vi "Week 3 Practical - CPitcel.vi"() -> ()   [LabVIEW 2018]
panel:
  out "Prime Result":string
  in  "Stop Operation":bool
  in  "Operation":string(combo)="Select Op"
  in  "Operand X":dbl
  in  "Operand Y":dbl
  out "Result":dbl
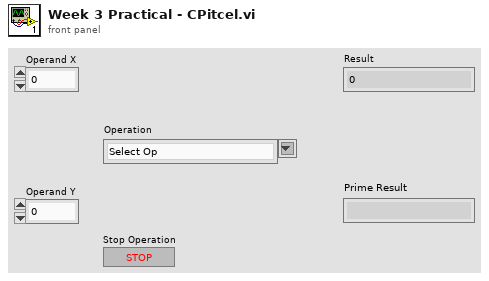
[diagram p1: front panel]
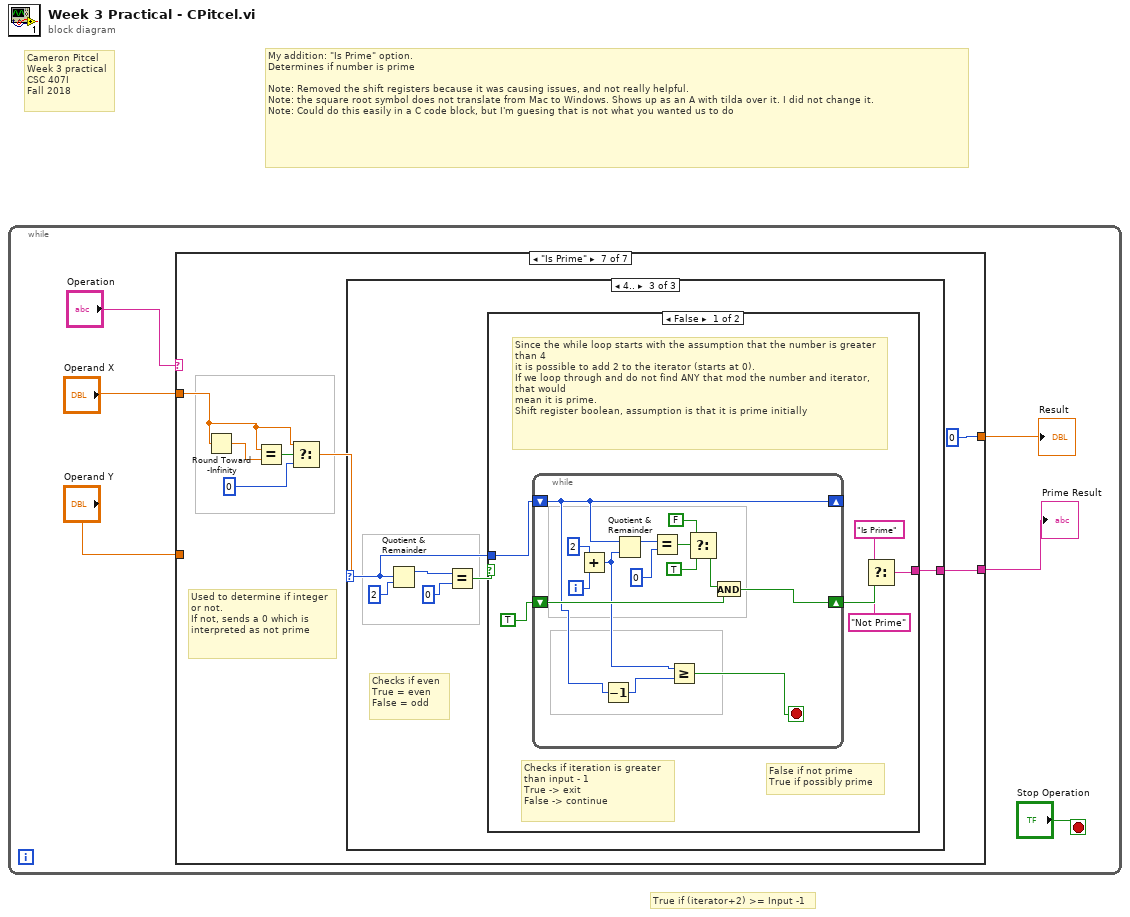
[diagram p0: block diagram]
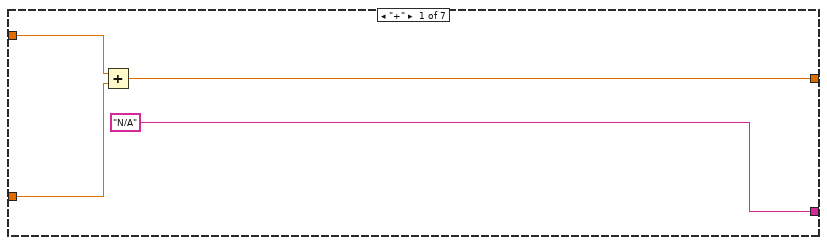
[diagram p2: hidden frame]
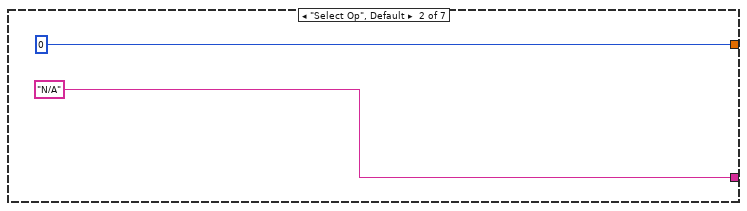
[diagram p3: hidden frame]
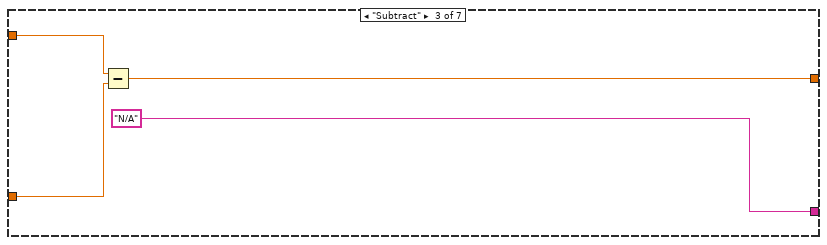
[diagram p4: hidden frame]
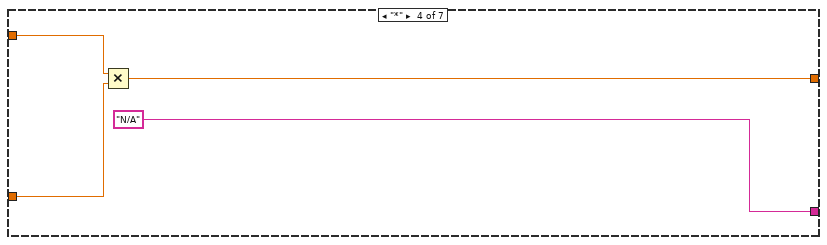
[diagram p5: hidden frame]
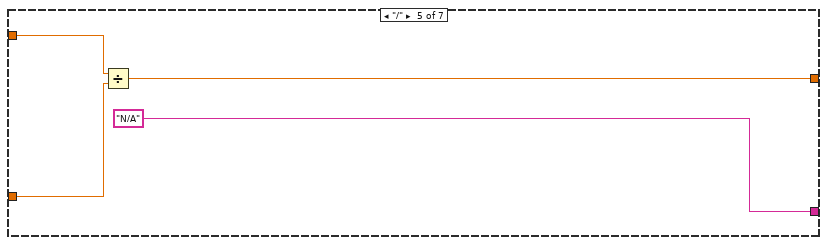
[diagram p6: hidden frame]
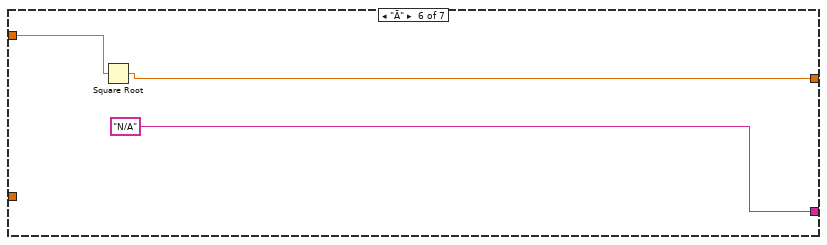
[diagram p7: hidden frame]
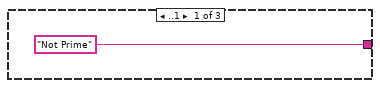
[diagram p8: hidden frame]
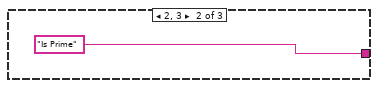
[diagram p9: hidden frame]
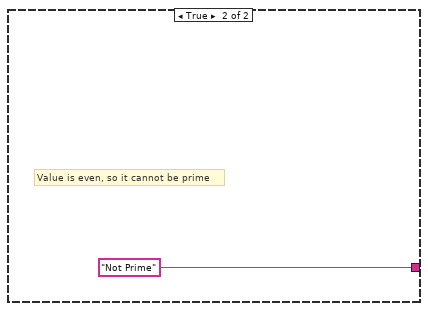
[diagram p10: hidden frame]
diagram:
  # "Cameron Pitcel\nWeek 3 practical\nCSC 407I\nFall 2018"
  # "True if (iterator+2) >= Input -1"
  # "My addition: \"Is Prime\" option.\nDetermines if number is prime\n\nNote: Removed the shift registers because it was causing issues, and not really helpful.\nNote: the square root symbol does not translate from Mac to Windows. Shows up as an A with tilda over it. I did not change it.\nNote: Could do this easily in a C code block, but I'm guesing that is not what you wanted us to do"
  n1 = while {
    stop <- "Stop Operation" stop-if-true
    n2 = case shown="\"Is Prime\"" "Operation" {
      tunnel: "Operand Y" -> [w9 _ w15 w19 w23 _ _]
      tunnel: "Operand X" -> [w10 _ w16 w20 w24 w27 w30]
      tunnel: [w8 0 w14 w18 w22 w26 0] -> w2
      tunnel: ["N/A" "N/A" "N/A" "N/A" "N/A" "N/A" w28] -> w1
      frame "+" {
        n3 = Add(x=w10, y=w9) -> (x+y=w8:dbl)
      }
      frame "Select Op", Default {
      }
      frame "Subtract" {
        n4 = Subtract(x=w16, y=w15) -> (x-y=w14:dbl)
      }
      frame "*" {
        n5 = Multiply(x=w20, y=w19) -> (x*y=w18:dbl)
      }
      frame "/" {
        n6 = Divide(x=w24, y=w23) -> (x/y=w22:dbl)
      }
      frame "Ã" {
        n7 = Square Root(x=w27) -> (sqrt(x)=w26:dbl)
      }
      frame "Is Prime" {
        # "Used to determine if integer or not.\nIf not, sends a 0 which is interpreted as not prime"
        n8 = Round Toward -Infinity(1:w30) -> (0:w33:dbl)
        n9 = Equal?(x=w30, y=w33) -> (x = y?=w31:bool)
        n10 = Select(t=w30, s=w31, f=0) -> (s? t:f=w32:dbl)
        n11 = case shown="4.." w32 {
          selector: w32 -> [_ _ w37]
          tunnel: ["Not Prime" "Is Prime" w39] -> w28
          frame ..1 {
          }
          frame 2, 3 {
          }
          frame 4.. {
            # "Checks if even\nTrue = even\nFalse = odd"
            n12 = Quotient & Remainder(x=w37, y=2) -> (x-y*floor(x/y)=w38:i32)  [unwired: 1 out]
            n13 = Equal?(x=w38, y=0) -> (x = y?=w40:bool)
            n14 = case shown="False" w40 {
              tunnel: [w44 "Not Prime"] -> w39
              tunnel: w37 -> [w48 _]
              frame False {
                # "Since the while loop starts with the assumption that the number is greater than 4\nit is possible to add 2 to the iterator (starts at 0).\nIf we loop through and do not find ANY that mod the number and iterator, that would \nmean it is prime.\nShift register boolean, assumption is that it is prime initially"
                # "Checks if iteration is greater \nthan input - 1\nTrue -> exit\nFalse -> continue"
                # "False if not prime\nTrue if possibly prime"
                n15 = while {
                  shift-right: [w51] -> _
                  shift-left: w48 -> [w51]
                  shift-right: [w53] -> w46
                  shift-left: TRUE -> [w54]
                  i -> [w62]
                  stop <- w49 stop-if-true
                  n16 = Add(x=2, y=w62) -> (x+y=w52:i32)
                  n17 = Decrement(x=w51) -> (x-1=w50:i32)
                  n18 = Quotient & Remainder(x=w51, y=w52) -> (x-y*floor(x/y)=w60:i32)  [unwired: 1 out]
                  n19 = Equal?(x=w60, y=0) -> (x = y?=w58:bool)
                  n20 = Greater Or Equal?(x=w52, y=w50) -> (x >= y?=w49:bool)
                  n21 = Select(t=FALSE, s=w58, f=TRUE) -> (s? t:f=w55:bool)
                  n22 = And(x=w55, y=w54) -> (x .and. y?=w53:bool)
                }
                n23 = Select(t="Is Prime", s=w46, f="Not Prime") -> (s? t:f=w44:string)
              }
              frame True {
                # "Value is even, so it cannot be prime"
              }
            }
          }
        }
      }
    }
    "Result" <- w2
    "Prime Result" <- w1
  }
